vi "Script.vi"(0 "entrée 1":dbl[](array[numeric]), 1 "entrée 2":dbl[](array[numeric]), 2 "pause":i32, 3 "C2":u32(colorbox)=8584960, 4 "entrée d'erreur":errorcluster, 5 "entrée 3":dbl[](array[numeric]), 6 "C3":u32(colorbox)=16754080, 7 "entrée 4":dbl[](array[numeric]), 9 "Seq":string) -> (20 "SCRIPT FINAL":string, 27 "sortie d'erreur":errorcluster)   [LabVIEW 2017]
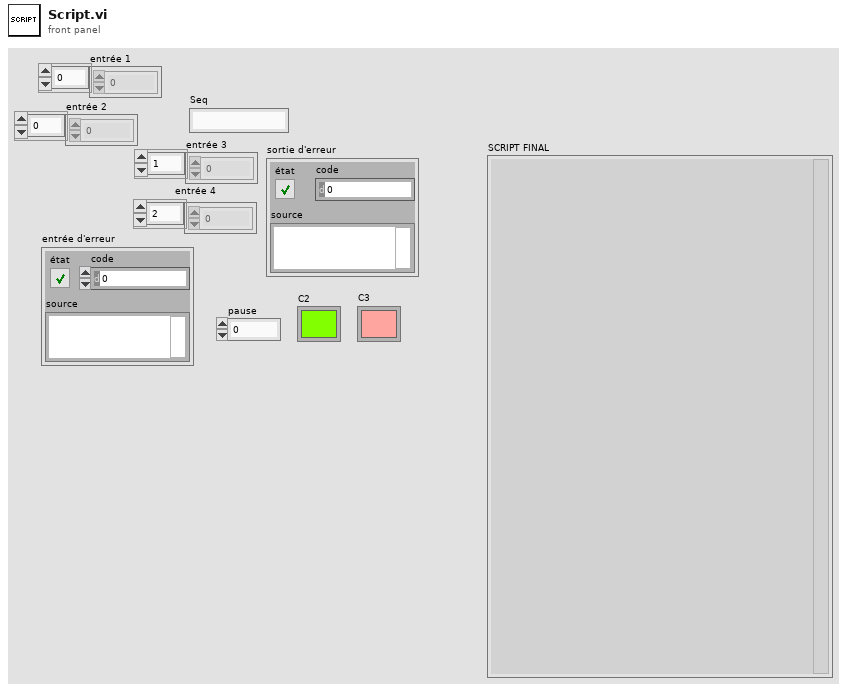
[diagram p1: front panel]
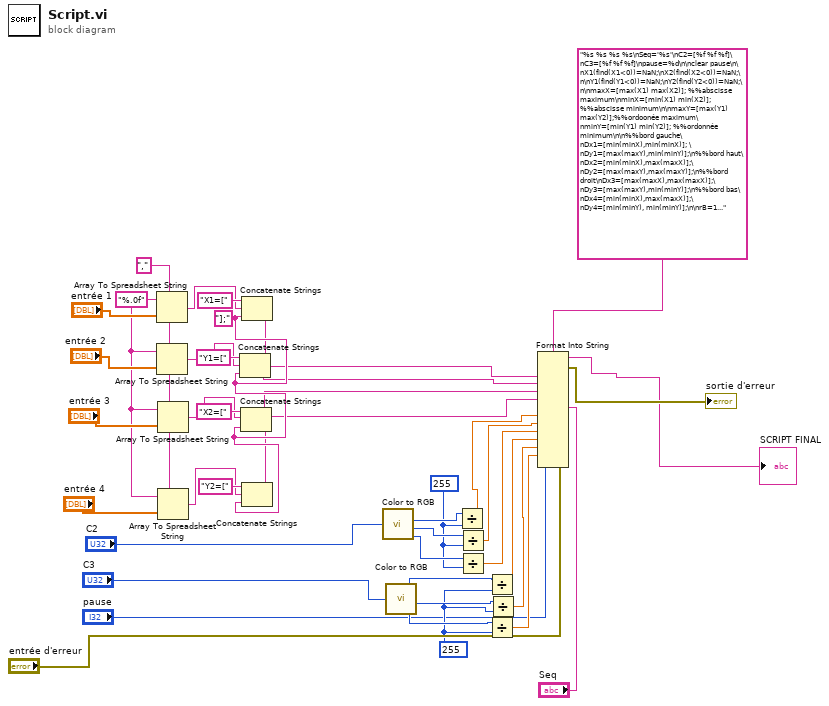
[diagram p0: block diagram]
diagram:
  w15 = 255
  w20 = u8 255 ("y")
  w27 = "];" ("chaîne")
  w26 = "," ("séparateur (Tabulation)")
  w25 = "%.0f" ("chaîne de format")
  n1 = Array To Spreadsheet String(delimiter (Tab)=w26, array="entrée 1", 3:w25) -> (spreadsheet string=w34:string)
  n2 = Array To Spreadsheet String(delimiter (Tab)=w26, array="entrée 2", 3:w25) -> (spreadsheet string=w30:string)
  n3 = Array To Spreadsheet String(delimiter (Tab)=w26, array="entrée 3", 3:w25) -> (spreadsheet string=w29:string)
  n4 = Array To Spreadsheet String(delimiter (Tab)=w26, array="entrée 4", 3:w25) -> (spreadsheet string=w28:string)
  n5 = Concatenate Strings("Y1=[" ("chaîne"), w30, w27) -> (w12:string)
  n6 = Concatenate Strings("X2=[" ("chaîne"), w29, w27) -> (w11:string)
  n7 = Concatenate Strings("X1=[" ("chaîne"), w34, w27) -> (w13:string)
  n8 = Concatenate Strings("Y2=[" ("chaîne"), w28, w27) -> (w10:string)
  n9 = call <vilib>:"Color to RGB.vi"("Color"="C2") -> ("R"=w23:u8, "G"=w22:u8, "B"=w21:u8)  [unwired: 1 out]
  n10 = call <vilib>:"Color to RGB.vi"("Color"="C3") -> ("R"=w18:u8, "G"=w17:u8, "B"=w16:u8)  [unwired: 1 out]
  n11 = Divide(x=w23, y=w20) -> (x/y=w7:dbl)
  n12 = Divide(x=w22, y=w20) -> (x/y=w6:dbl)
  n13 = Divide(x=w21, y=w20) -> (x/y=w5:dbl)
  n14 = Divide(x=w18, y=w15) -> (x/y=w4:dbl)
  n15 = Divide(x=w16, y=w15) -> (x/y=w2:dbl)
  n16 = Divide(x=w17, y=w15) -> (x/y=w3:dbl)
  n17 = Format Into String(format string="%s %s %s %s\nSeq='%s'\nC2=[%f %f %f]\nC3=[%f %f %f]\npause=%d\n\nclear pause\n\nX1(find(X1<0))=NaN;\nX2(find(X2<0))=NaN;\n\nY1(find(Y1<0))=NaN;\nY2(find(Y2<0))=NaN;\n\nmaxX=[max(X1) max(X2)]; %%abscisse maximum\nminX=[min(X1) min(X2)]; %%abscisse minimum\n\nmaxY=[max(Y1) max(Y2)];%%ordoonée maximum\nminY=[min(Y1) min(Y2)]; %%ordonnée minimum\n\n%%bord gauche\nDx1=[min(minX),min(minX)]; \nDy1=[max(maxY),min(minY)];\n%%bord haut\nDx2=[min(minX),max(maxX)];\nDy2=[max(maxY),max(maxY)];\n%%bord droit\nDx3=[max(maxX),max(maxX)];\nDy3=[max(maxY),min(minY)];\n%%bord bas\nDx4=[min(minX),max(maxX)];\nDy4=[min(minY), min(minY)];\n\nrB=15;\nZ=0;\n\n%%La distance limite et changement d'angle minimum pour que ce soit un choc sont fixés\n\ndmin=50;\nalphamin=1;\n\n%%On calcule la distance entre les pucks\n%%Création d'un vecteur de booléens avec \"true\" si la distance est inférieure à dmin\n%%En multipliant par un vecteur d'indexes, on obtient un vecteur avec des index s'il y a un choc potentiel et zero s'il n'y en a pas\n\nDistancePucks=sqrt((X1-X2).^2+(Y1-Y2).^2);\nt=DistancePucks<dmin;\nConditionDistance=t.*(1:length(X1));\n\n%%Changement de direction\n%%Différence entre 2 éléments des vecteurs positions pour calculer la pente (tangente de l'angle par rapport à l'horizontale)\nX1Diff=diff(X1);\nY1Diff=diff(Y1);\nAngles1=atan2(Y1Diff,X1Diff);\nX2Diff=diff(X2);\nY2Diff=diff(Y2);\nAngles2=atan2(Y2Diff,X2Diff);\n\nA=abs(diff(Angles1));\nB=abs(diff(Angles2));\n\n%%On cherche les positions où à la fois le puck 1 et 2 ont une variation d'angle de plus de 1 radian\nC=find(A>alphamin | B>alphamin); %%opérateur logique \"ou\"\n\n%%Le vecteur C nous donne la position avant le changement de trajectoire, nous cherchons donc celle d'après: il faut l'incrémenter de 1\n\nConditionAngle=C+1;\n\n%%Le choc se produit si les deux conditions décrites sont satisfaites simultanément\n\nConditionChoc=intersect(ConditionAngle,ConditionDistance);\n\n%%On ne valide que les chocs  partir du 11e index afin d'éviter que le début ne soit interprété comme une succession de chocs (les pucks viennent d'être déposés sur la table)\n\nchoc=ConditionChoc(find(ConditionChoc>10));\n\n%%Détection des rebonds premier puck\n\n%%Bord droit\nBD1=find((max(maxX)-X1)<=rB);\nBD1(1+find(diff(BD1)==1))=[];\n\n%%Bord gauche\nBG1=find((X1-min(minX))<=rB);\nBG1(1+find(diff(BG1)==1))=[];\n\n%%Bord haut\nBH1=find((Y1+rB)>=max(maxY));\nBH1(1+find(diff(BH1)==1))=[];\n\n%%Bord bas\nBB1=find((Y1-rB)<=min(minY));\nBB1(1+find(diff(BB1)==1))=[];\n\n%%Détection des rebonds deuxième puck\n\n%%Bord droit\nBD2=find((max(maxX)-X2)<=rB);\nBD2(1+find(diff(BD2)==1))=[];\n\n%%Bord gauche\nBG2=find((X2-min(minX))<=rB);\nBG2(1+find(diff(BG2)==1))=[];\n\n%%Bord haut\nBH2=find((Y2+rB)>=max(maxY));\nBH2(1+find(diff(BH2)==1))=[];\n\n%%Bord bas\nBB2=find((Y2-rB)<=min(minY));\nBB2(1+find(diff(BB2)==1))=[];\n\n\nfig=figure('Name','Air Hockey');\nhold on\n\nplot(Dx1,Dy1,'k',Dx2,Dy2,'k',Dx3,Dy3,'k',Dx4,Dy4,'k','linewidth',0.5);\naxis([min(minX)-30 max(maxX)+50 min(minY)-60 max(maxY)+30]);\n\np1=plot(X1,Y1,'-o','markerfacecolor',[C2(1) C2(2) C2(3)]);\np2=plot(X2,Y2,'-o','markerfacecolor',[C3(1) C3(2) C3(3)]);\np1.Color=[C2(1) C2(2) C2(3)]; \np2.Color=[C3(1) C3(2) C3(3)]; %%on applique les couleurs choisies depuis Labview\n\nscatter([X1(choc),X2(choc)],[Y1(choc),Y2(choc)],2000,'markerfacecolor','r','markeredgecolor','r','markerfacealpha',0.2,'linewidth',1); %%choix des paramètres de \"décoration\" du point de choc entre les pucks\nscatter(X1([BD1,BG1,BH1,BB1]),Y1([BD1,BG1,BH1,BB1]),400,'markeredgecolor',[C2(1) C2(2) C2(3)]);\nscatter(X2([BD2,BG2,BH2,BB2]),Y2([BD2,BG2,BH2,BB2]),400,'markeredgecolor',[C3(1) C3(2) C3(3)]);\n\ntext((min(minX)+max(maxX))/2-30,max(maxY)+50,'Air Hockey','Color','black','FontSize',14,'FontWeight','bold');%%affichage du titre\nxlabel ('Largeur');\nylabel ('Hauteur');\n\ntext(30,max(maxY)+20,Seq); %%Seq provient de LabView, c'est un string qui vaut soit 'Seq1m', soit 'Seq2m'\nt=datetime('now');\ntext(30+60,max(maxY)+20,datestr(t)); %%affichage de date et heure actuelles\n\nstr1=\"%%i bands hit by puck 1\";\ntxt1=length(BD1)+length(BG1)+length(BH1)+length(BB1);\nlegende1=sprintf(str1,txt1);\n\nstr2=\"%%i bands hit by puck 2\";\ntxt2=length(BD2)+length(BG2)+length(BH2)+length(BB2);\nlegende2=sprintf(str2,txt2);\n\nstr3=\"%%i puck collision(s)\";\ntxt3=length(choc);\nlegende3=sprintf(str3,txt3);\n\ntext(min(minX),min(minY)-15,legende1);%%affichage du nombre de chocs entre puck1 et bandes\ntext(min(minX),min(minY)-25,legende2);%%affichage du nombre de chocs entre puck2 et bandes\ntext(min(minX),min(minY)-35,legende3);%%affichage du nombre de collisions entre pucks\n\n\nhold off\nsaveas(fig,'AH_score','pdf') %%sauvegarde du document PDF\n%%saveas est placé ici car dans le cas où l'on viendrait à fermer la fenêtre avant que le temps de valeur pause ne s'écoule, le fichier serait créé de toute façon\n\nclear all\npause(10);\n\n\n" ("chaîne de format"), error in="entrée d'erreur", w13, w12, w11, w10, "Seq", w7, w6, w5, w4, w3, w2, "pause") -> (resulting string=→"SCRIPT FINAL":string, error out=→"sortie d'erreur":errorcluster)  [unwired: 1 in]
